vi "Measure.vi"(6 "Init work":bool, 7 "Update period":dbl, 8 "error in (no error)":errorcluster, 9 "Last request":bool, 10 "Requester":string, 11 "Resonance Detector in":refnum<class "Resonance Detector.lvclass">) -> (0 "error out":errorcluster, 3 "Resonance Detector out":refnum<class "Resonance Detector.lvclass">)   [LabVIEW 2024, in "Resonance Detector.lvclass"]
uses:
  Resonance Detector.lvclass
  Resonance Detector.lvclass/Resonance Detector.ctl
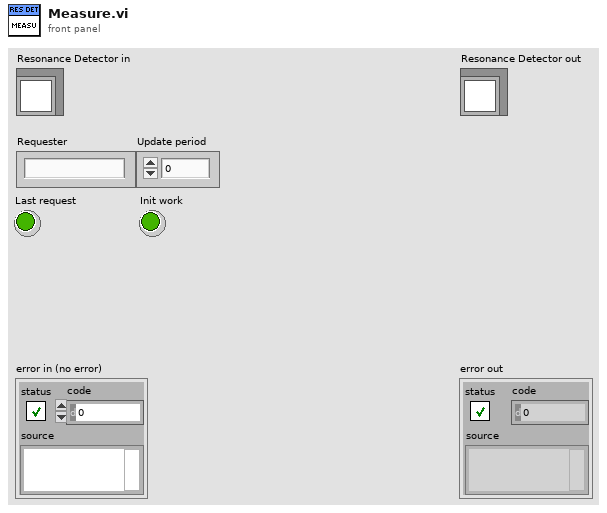
[diagram p1: front panel]
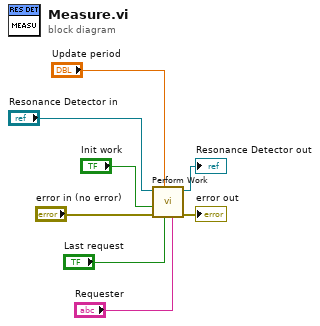
[diagram p0: block diagram]
diagram:
  n1 = call-dynamic "Perform Work.vi"("Controller name"="Requester", "Last request"="Last request", "Update period"="Update period", "error in (no error)"="error in (no error)", "Initialize"="Init work", "Measure Object in"="Resonance Detector in") -> ("error out"=→"error out":errorcluster, "Measure Object out"=→"Resonance Detector out":refnum<class "Resonance Detector.lvclass">)  [unwired: 4 in]
